vi "NI ELVIS - Close Wrap.vi"(8 "error in":errorcluster, 11 "NI ELVIS Refnum In":T1) -> (0 "error out":errorcluster)   [LabVIEW 2012]
uses:
  <instrlib>/NI ELVIS Traditional/NI ELVIS - RSCMAN.llb/ELVIS RSCMAN - NI ELVIS Refnum.ctl
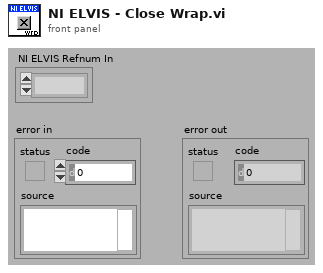
[diagram p1: front panel]
types:
  T1 = typedef "ELVIS RSCMAN - NI ELVIS Refnum.ctl" = refnum<k1>
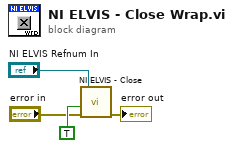
[diagram p0: block diagram]
diagram:
  n1 = call <instrlib>:"NI ELVIS - Close.vi"("error in"="error in", "Clear Routing?"=TRUE, "NI ELVIS Refnum In"="NI ELVIS Refnum In") -> ("error out"=→"error out":errorcluster)  [unwired: 4 in]
